vi "N4_X01_WriteAndCheck.vi"(4 "Driver Name":T9, 5 "Command Time (s)":T6=3.0, 6 "Error Code":T10, 7 "Command":T7, 8 "error in":T8, 11 "DriverConnect in":T1={"InterfaceType"=enum."VISA", "OpenedSession"="", "InterfaceSettings"={"Interface"=enum."RS232", "EOS 4 read"=enum."LF (\\n)", "EOS 4 write"=enum."LF (\\n)", "TMO, ms"=10000, "Sett"=variant(cluster{"Baud Rate":u32, "Data Bits":u16, "Parity":u16, "Stop Bits":u16, "Flow Control":u16, "Eho":bool} {"Baud Rate"=75, "Data Bits"=0, "Parity"=0, "Stop Bits"=0, "Flow Control"=0, "Eho"=FALSE})}}) -> (0 "error out":T8, 3 "DriverConnect out":T1={"InterfaceType"=enum."VISA", "OpenedSession"="", "InterfaceSettings"={"Interface"=enum."RS232", "EOS 4 read"=enum."LF (\\n)", "EOS 4 write"=enum."LF (\\n)", "TMO, ms"=10000, "Sett"=variant(cluster{"Baud Rate":u32, "Data Bits":u16, "Parity":u16, "Stop Bits":u16, "Flow Control":u16, "Eho":bool} {"Baud Rate"=75, "Data Bits"=0, "Parity"=0, "Stop Bits"=0, "Flow Control"=0, "Eho"=FALSE})}})   [LabVIEW 2018]
uses:
  MOKO_LabViewLibrary/MokoLowLevel/MokoLowLovelControl/MLLC_ErrorCode.ctl
  MOKO_LabViewLibrary/MokoLowLevel/MokoLowLovelControl/MLLC_DriverName.ctl
  MOKO_LabViewLibrary/MokoLowLevel/MokoLowLovelControl/MLLC_Error.ctl
  MOKO_LabViewLibrary/MokoLowLevel/MokoLowLovelControl/MLLC_Command.ctl
  MOKO_LabViewLibrary/MokoLowLevel/MokoLowLovelControl/MLLC_Delay.ctl
  MOKO_LabViewLibrary/MokoLowLevel/MokoLowLovelControl/MLLC_ConnectCluster.ctl
  MOKO_LabViewLibrary/MokoLowLevel/MokoLowLovelControl/MLLC_InterfaceType.ctl
  MOKO_LabViewLibrary/MokoLowLevel/MokoLowLovelControl/MLLC_OpenedSession.ctl
  MOKO_LabViewLibrary/MokoLowLevel/MokoLowLovelControl/MLLC_InterfaceSettings.ctl
  MOKO_LabViewLibrary/MokoLowLevel/MokoLowLovelControl/MLLC_InterfaceKind.ctl
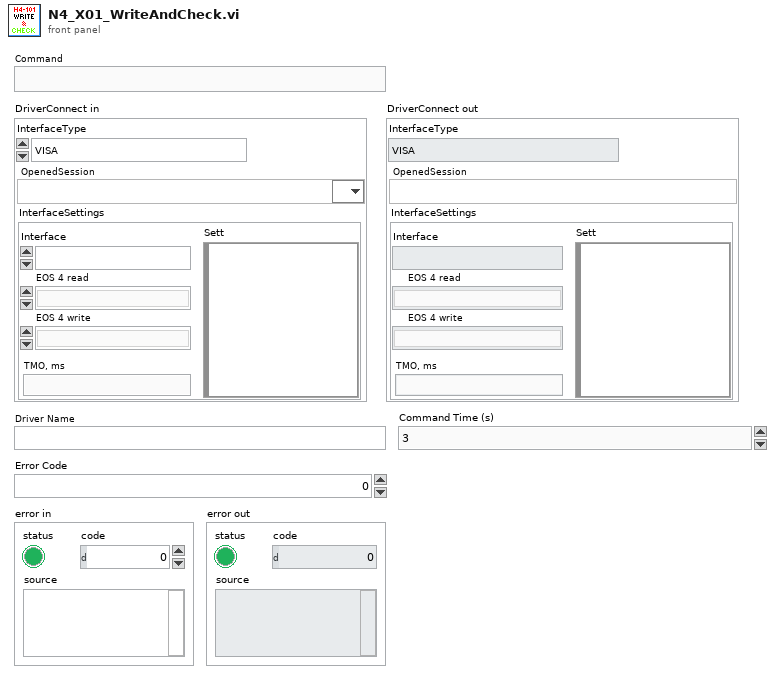
[diagram p1: front panel]
types:
  T1 = typedef "MLLC_ConnectCluster.ctl" = cluster{"InterfaceType":T2, "OpenedSession":T3, "InterfaceSettings":T4}
  T2 = typedef "MLLC_InterfaceType.ctl" = enum16{"VISA", "Prologix USB-GPIB"}
  T3 = typedef "MLLC_OpenedSession.ctl" = refnum<visa-resource-name>
  T4 = typedef "MLLC_InterfaceSettings.ctl" = cluster{"Interface":T5, "EOS 4 read":enum16{"Default (=EOS 4 write)", "CR (\\r)", "LF (\\n)", "None"}, "EOS 4 write":enum16{"CR+LF (\\r\\n)", "CR (\\r)", "LF (\\n)", "None"}, "TMO, ms":i32, "Sett":variant}
  T5 = typedef "MLLC_InterfaceKind.ctl" = enum16{"RS232", "GPIB", "USB", "Ethernet", "another"}
  T6 = typedef "MLLC_Delay.ctl" = dbl
  T7 = typedef "MLLC_Command.ctl" = string
  T8 = typedef "MLLC_Error.ctl" = errorcluster
  T9 = typedef "MLLC_DriverName.ctl" = string
  T10 = typedef "MLLC_ErrorCode.ctl" = u32
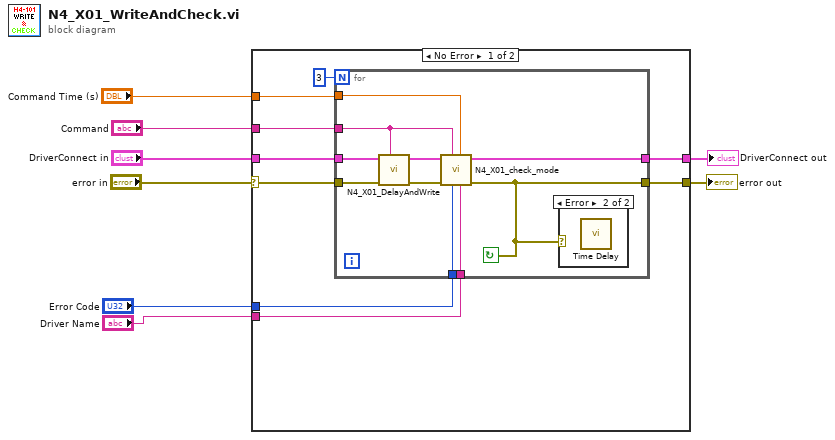
[diagram p0: block diagram]
diagram:
  n1 = case shown="No Error" "error in" {
    selector: "error in" -> [w11 w29]
    tunnel: [w12 w29] -> w8
    tunnel: [w13 w28] -> w1
    tunnel: "Error Code" -> [w15 _]
    tunnel: "Driver Name" -> [w14 _]
    tunnel: "DriverConnect in" -> [w16 w28]
    tunnel: "Command" -> [w17 _]
    tunnel: "Command Time (s)" -> [w10 _]
    frame No Error {
      n2 = for {
        N: 3 -> [_]
        tunnel: w17 -> [w26]
        tunnel: w16 -> [w25]
        tunnel: w15 -> [w24]
        tunnel: w14 -> [w23]
        tunnel: [w22] -> w13
        tunnel: [w18] -> w12
        tunnel: w11 -> [w20]
        tunnel: w10 -> [w19]
        stop <- w18 continue-if-true
        n3 = call "N4_X01_DelayAndWrite.vi"("Command"=w26, "error in"=w20, "DriverConnect in"=w25) -> ("error out"=w21:T8, "DriverConnect out"=w27:T1)  [unwired: 7 in]
        n4 = call "N4_X01_check_mode.vi"("Driver Name"=w23, "Delay befor,s"=w19, "Error Code"=w24, "InputParam"=w26, "error in"=w21, "DriverConnect in"=w27) -> ("error out"=w18:T8, "DriverConnect out"=w22:T1)  [unwired: 4 in]
        n5 = case shown="Error" w18 {
          frame No Error {
          }
          frame Error {
            n6 = call "Time Delay"() -> ()  [unwired: 11 in, 1 out]
          }
        }
      }
    }
    frame Error {
    }
  }
  "error out" <- w8
  "DriverConnect out" <- w1
